vi "RZ bipolar.vi"() -> ()   [LabVIEW 2014]
uses:
  <vilib>/Analysis/NI_AALPro.lvlib
panel:
  out "Waveform Chart 3":dbl[](graph)
  out "Waveform Chart 2":i16[](graph)
  in  "Numeric":i32
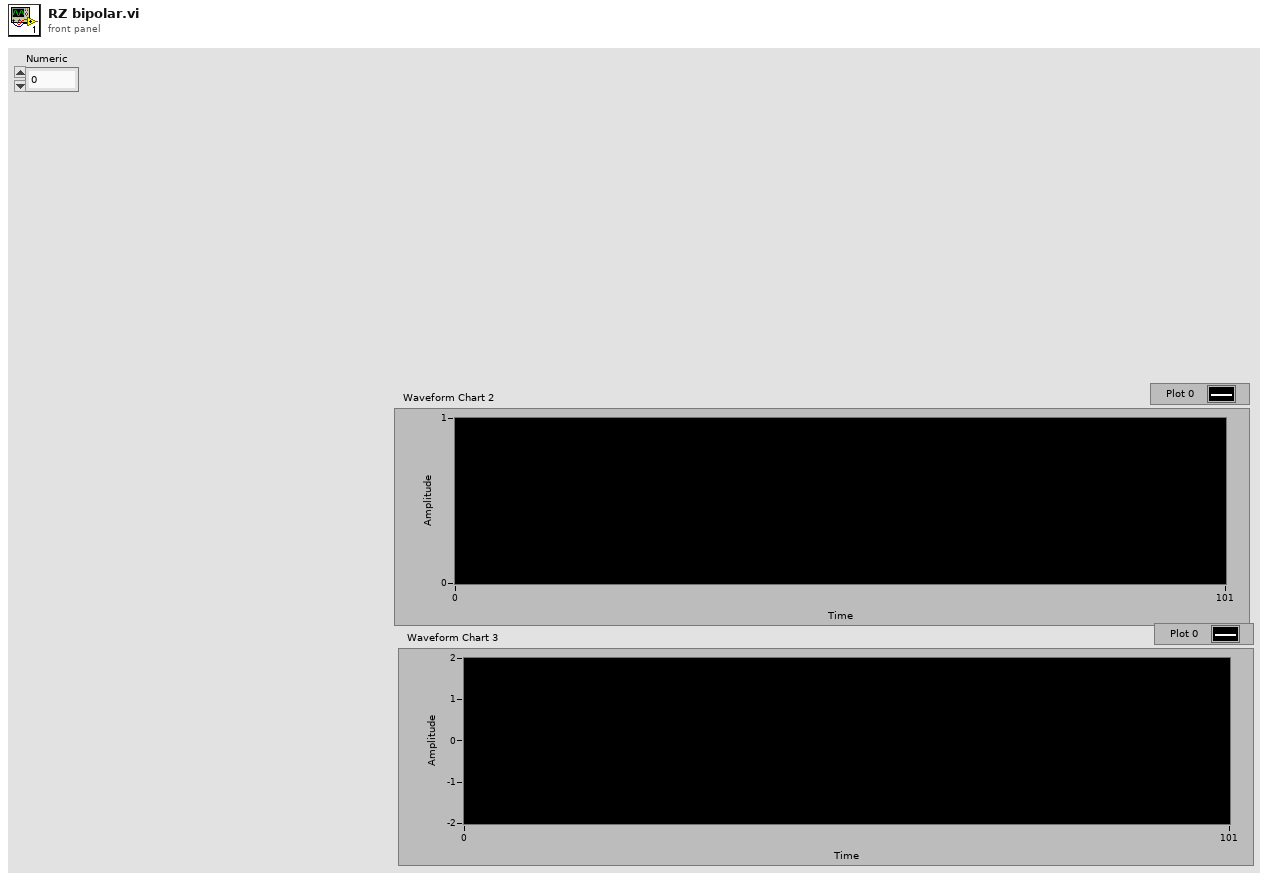
[diagram p1: front panel]
types:
  T1 = enum16{"sine", "cosine", "triangle", "square", "sawtooth", "increasing ramp", "decreasing ramp"}
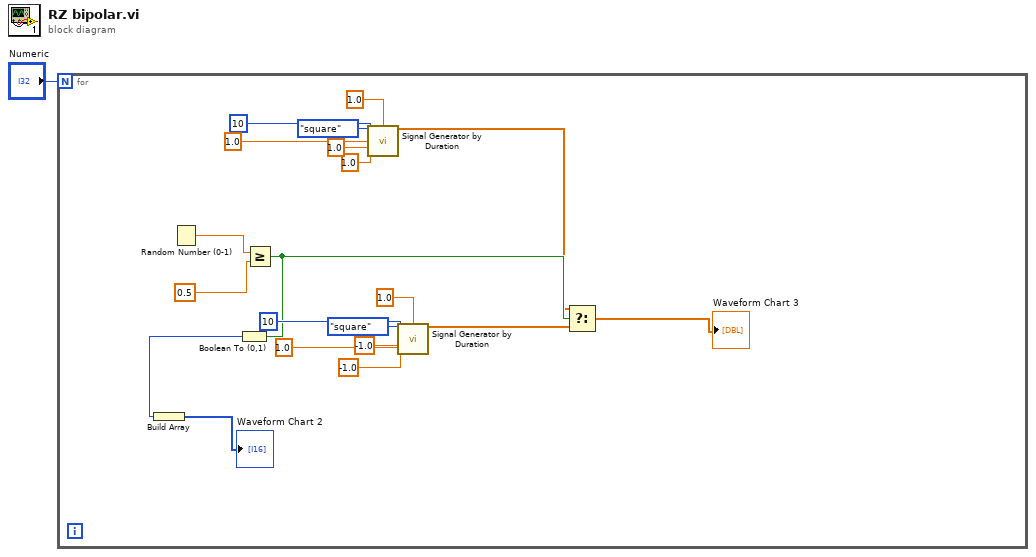
[diagram p0: block diagram]
diagram:
  n1 = for {
    N: "Numeric" -> [_]
    n2 = Random Number (0-1)() -> (number: 0 to 1=w21:dbl)
    n3 = Greater Or Equal?(x=w21, y=0.5) -> (x >= y?=w5:bool)
    n4 = Boolean To (0,1)(Boolean=w5) -> (0, 1=w19:i16)
    n5 = Build Array(w19) -> (→"Waveform Chart 2":i16[])
    n6 = call <vilib>:"Signal Generator by Duration.vi"("signal type"=T1."square", "duration"=1.0, "# of samples"=10, "frequency"=1.0, "amplitude"=1.0, "dc offset"=1.0) -> ("signal"=w3:dbl[])  [unwired: 6 in, 3 out]
    n7 = call <vilib>:"Signal Generator by Duration.vi"("signal type"=T1."square", "duration"=1.0, "# of samples"=10, "frequency"=1.0, "amplitude"=-1.0, "dc offset"=-1.0) -> ("signal"=w2:dbl[])  [unwired: 6 in, 3 out]
    n8 = Select(t=w3, s=w5, f=w2) -> (s? t:f=→"Waveform Chart 3":dbl[])
  }
